vi "One button pneumatic.vi"(6 "Prev State In":bool, 8 "State In":bool, 11 "Input 1":bool) -> (0 "State Out":bool, 2 "Output 2":bool, 3 "Output 1":bool, 4 "Prev State Out":bool)   [LabVIEW 2014]
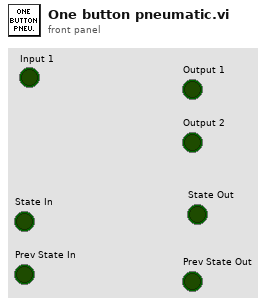
[diagram p1: front panel]
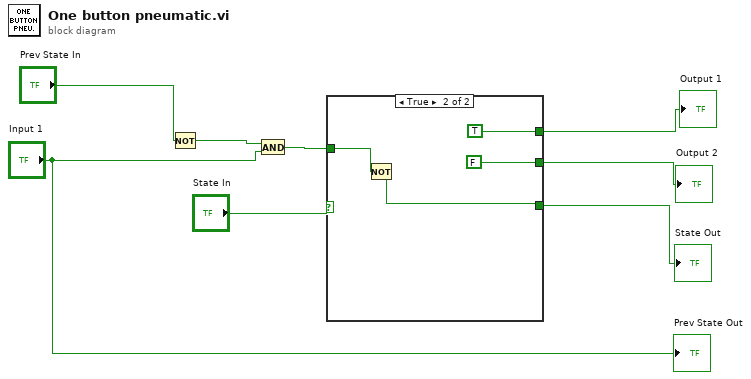
[diagram p0: block diagram]
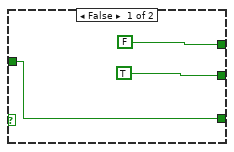
[diagram p2: hidden frame]
diagram:
  n1 = Not(x="Prev State In") -> (.not. x?=w8:bool)
  n2 = And(x=w8, y="Input 1") -> (x .and. y?=w3:bool)
  n3 = case shown="True" "State In" {
    tunnel: [FALSE TRUE] -> w7
    tunnel: [TRUE FALSE] -> w6
    tunnel: [w9 w13] -> w5
    tunnel: w3 -> [w9 w12]
    frame False {
    }
    frame True {
      n4 = Not(x=w12) -> (.not. x?=w13:bool)
    }
  }
  "Output 1" <- w7
  "Output 2" <- w6
  "State Out" <- w5
  "Prev State Out" <- "Input 1"
